vi "Extreme Value PDF.vi"(9 "b":dbl=1.0, 10 "a":dbl, 11 "x":dbl) -> (0 "error":i32, 3 "pdf(x)":dbl=0.36787944117144233)   [LabVIEW 2010, in "NI_Gmath.lvlib"]
doc: "Computes the continuous probability density function (PDF) of various distributions. You must manually select the polymorphic instance to use."
uses:
  NI_Gmath.lvlib
  st_error_code.ctl
panel:
  # "Extreme Value PDF"
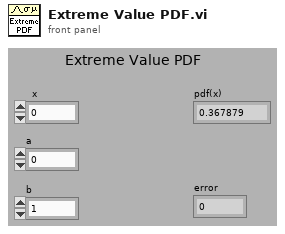
[diagram p1: front panel]
types:
  T1 = typedef "NI_Gmath.lvlib/st_error_code.ctl" = i32
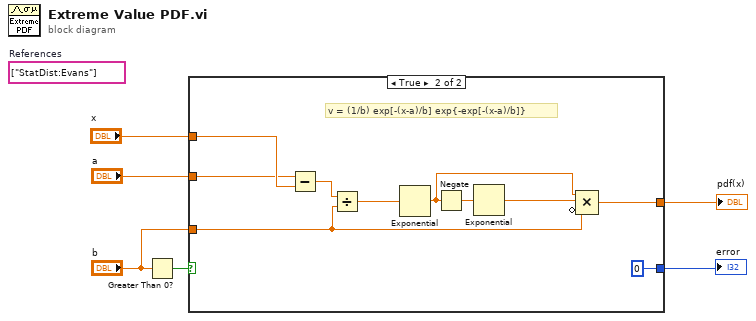
[diagram p0: block diagram]
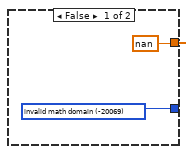
[diagram p2: hidden frame]
diagram:
  (unwired) string[] ["StatDist:Evans"]  # References
  n1 = Greater Than 0?(x="b") -> (x > 0?=w2:bool)
  n2 = case shown="True" w2 {
    tunnel: "b" -> [_ w13]
    tunnel: [w7 0 ("invalid math domain")] -> w6
    tunnel: [nan w10] -> w5
    tunnel: "x" -> [_ w17]
    tunnel: "a" -> [_ w16]
    frame False {
      w7 = T1 -20069 items=["invalid math domain"=-20069, "Fourier interpolation size m >= n"=-20070, "empty array"=-20003] ("stat interp error code")
    }
    frame True {
      # "v = (1/b) exp[-(x-a)/b] exp{-exp[-(x-a)/b]}"
      n3 = Subtract(x=w16, y=w17) -> (x-y=w15:dbl)
      n4 = Divide(x=w15, y=w13) -> (x/y=w9:dbl)
      n5 = Exponential(1:w9) -> (0:w11:dbl)
      n6 = Negate(x=w11) -> (-x=w14:dbl)
      n7 = Exponential(1:w14) -> (0:w12:dbl)
      n8 = Compound Arithmetic op=MULTIPLY(w11, w12, invert w13) -> (w10:dbl)
    }
  }
  "pdf(x)" <- w5
  "error" <- w6
